vi "fpga_ResamlingCore (32ch).vi"(0 "data in":i32, 1 "Channel number":u8, 2 "timestamp":fxp<+,64,32> format="%.42g", 5 "input data valid":bool, 7 "reference in":fxp<+/-,24,3>, 9 "input reference valid":bool, 11 "interpolation factor":u16=192, 12 "Ready for output":bool, 13 "Fnom":T1 items=["Fnom=50Hz", "Fnom=60Hz"]) -> (4 "Resample data and time":T2, 8 "resampling valid":bool, 10 "output valid":bool, 14 "Ready for reference input":bool, 15 "FIFO timeout?":bool)   [LabVIEW 2014, in "NI_EP_Resample_FPGA.lvlib"]
uses:
  <vilib>/addons/Electrical Power/PQ/Resampling/NI_EP_Resample_FPGA.lvlib
  <vilib>/addons/Electrical Power/PQ/Resampling/FPGA/subVIs/fpga_Resampled.ctl
  <vilib>/addons/Electrical Power/PQ/Resampling/FPGA/subVIs/fpga_Typedef Fnom.ctl
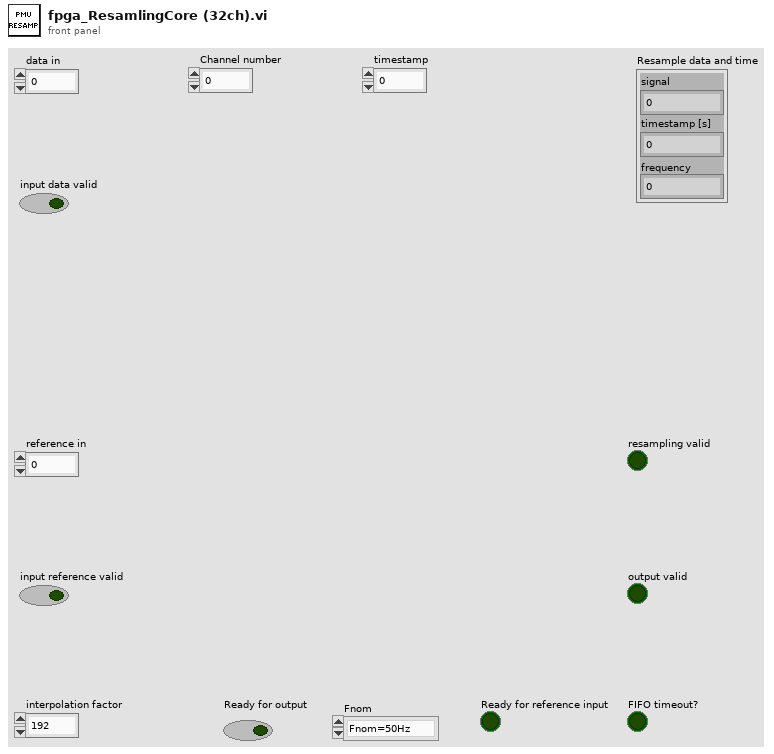
[diagram p1: front panel]
types:
  T1 = typedef "NI_EP_Resample_FPGA.lvlib/fpga_Typedef Fnom.ctl" = u8
  T2 = typedef "NI_EP_Resample_FPGA.lvlib/fpga_Resampled.ctl" = cluster{"signal":fxp<+/-,32,3>, "timestamp [s]":fxp<+,64,32>, "frequency":fxp<+,32,8>}
  T3 = cluster{"bufsize":u16, "bufsize-1":u16, "NChan":u8, "NChan-1":u8, "1/2SymPeriods":i8, "Neg1/2SymPeriods":i8, "polyOrder-1":u8, "maxDec-1":u8}
  T4 = cluster{"TAI timestamp":fxp<+,64,32>, "AI Count":u16}
  T5 = cluster{"even-angle signal":fxp<+/-,32,3>, "Resample position":fxp<+,64,16>, "frequency":fxp<+,32,8>}
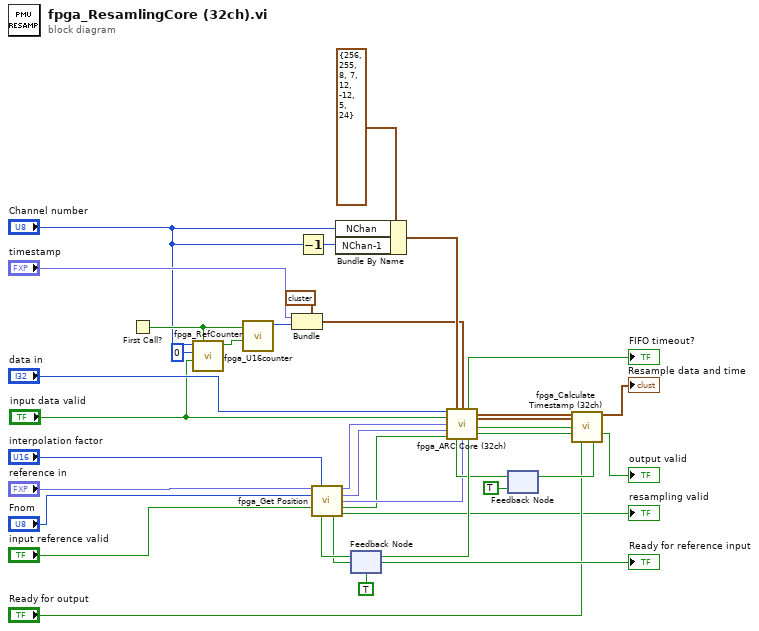
[diagram p0: block diagram]
diagram:
  n1 = First Call?() -> (First Call?: T/F=w14:bool)
  n2 = call <vilib>:"fpga_RefCounter.vi"("reset"=w14, "input valid?"="input data valid", "Reference index"=u8 0, "NChan"="Channel number") -> ("Multichannel enable"=w15:bool)  [unwired: 6 in, 1 out]
  n3 = call <vilib>:"fpga_U16counter.vi"("input valid"=w15, "reset"=w14) -> ("Counter"=w8:u16)  [unwired: 9 in]
  n4 = Bundle(cluster=T4 {"TAI timestamp"=0.0, "AI Count"=0} ("Time count"), "TAI timestamp"="timestamp", "AI Count"=w8) -> (w2:T4)
  n5 = Decrement(x="Channel number") -> (x-1=w17:u8)
  n6 = Bundle By Name(cluster=T3 {"bufsize"=256, "bufsize-1"=255, "NChan"=8, "NChan-1"=7, "1/2SymPeriods"=12, "Neg1/2SymPeriods"=-12, "polyOrder-1"=5, "maxDec-1"=24} ("ARC Constants"), "NChan"="Channel number", "NChan-1"=w17) -> (w11:T3)
  n7 = feedback #1(TRUE ("ready for input")) -> (w33:bool)
  n8 = call <vilib>:"fpga_Get Position.vi"("tach input"="reference in", "Interpolation factor"="interpolation factor", "Fnom"="Fnom", "input valid"="input reference valid", "ready for output"=w33) -> ("resample position [U64.16]"=w27:fxp<+,64,16>, "stepsize [U64.8]"=w28:fxp<+,64,8>, "frequency"=w9:fxp<+,32,8>, "output valid"=w3:bool, "Ready for input"=→"Ready for reference input":bool, "resampling valid"=→"resampling valid":bool)  [unwired: 5 in]
  n9 = feedback #2(TRUE ("ready for input")) -> (w23:bool)
  n10 = call <vilib>:"fpga_ARC Core (32ch).vi"("data input"="data in", "ARC Constants"=w11, "timestamp&count"=w2, "data valid"="input data valid", "resample position [U64.16]"=w27, "stepsize [U64.8]"=w28, "position valid"=w3, "Ready for output"=w23, "Frequency"=w9) -> ("FIFO timeout?"=→"FIFO timeout?":bool, "resample data"=w26:T5, "timestamp&count"=w1:T4, "muti_ch position valid?"=w4:bool, "ready for input"=w34:bool, "output valid"=w25:bool)  [unwired: 1 in]
  n11 = feedback-in #1(w34) -> ()
  n12 = call <vilib>:"fpga_Calculate Timestamp (32ch).vi"("resample data and position"=w26, "timestamp&count"=w1, "muti_ch position valid?"=w4, "input valid"=w25, "ready for output"="Ready for output") -> ("Resample data and time"=→"Resample data and time":T2, "output valid"=→"output valid":bool, "ready for input"=w24:bool)  [unwired: 8 in]
  n13 = feedback-in #2(w24) -> ()
